vi "AfterSamePositionColor-V2.2.vi"(3 "WhichPlayer":i32, 4 "index (col)":i32, 5 "index (row)":i32, 6 "BackMap":i32[][](array[numeric])) -> (2 "Numeric":dbl)   [LabVIEW 2014]
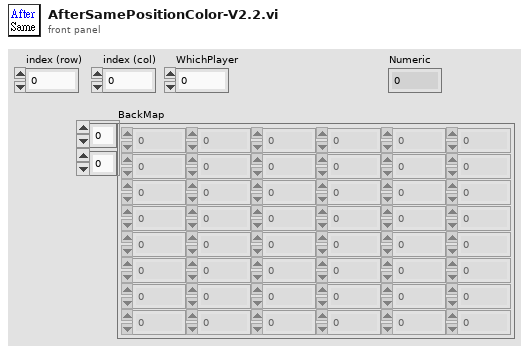
[diagram p1: front panel]
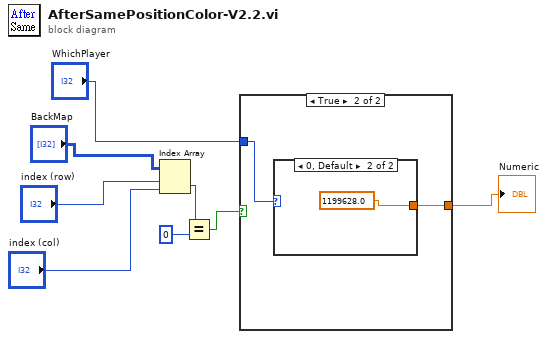
[diagram p0: block diagram]
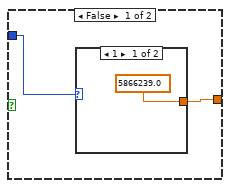
[diagram p2: hidden frame]
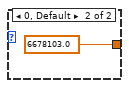
[diagram p3: hidden frame]
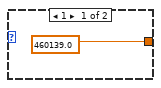
[diagram p4: hidden frame]
diagram:
  n1 = Index Array(array="BackMap", index (row)="index (row)", index (col)="index (col)") -> (element=w8:i32)
  n2 = Equal?(x=w8, y=0) -> (x = y?=w6:bool)
  n3 = case shown="True" w6 {
    tunnel: [w10 w14] -> w2
    tunnel: "WhichPlayer" -> [w9 w13]
    frame False {
      n4 = case shown="1" w9 {
        tunnel: [5866239.0 6678103.0] -> w10
        frame 1 {
        }
        frame 0, Default {
        }
      }
    }
    frame True {
      n5 = case shown="0, Default" w13 {
        tunnel: [460139.0 1199628.0] -> w14
        frame 1 {
        }
        frame 0, Default {
        }
      }
    }
  }
  "Numeric" <- w2
